vi "sub vi - Move Piezo Stage (Single).vi"(3 "frequency":dbl=0.5 min=0.0, 4 "Desired Position (um)":dbl min=0.0 format="%0.6f", 5 "Axis":u16(ring) items=["X", "Y", "Z"]) -> (0 "Z Position":dbl, 1 "Y Position":dbl, 2 "X Position":dbl)   [LabVIEW 2010]
uses:
  <vilib>/DAQmx/write.llb/DAQmx Write (Analog DBL 1Chan 1Samp).vi
  <vilib>/DAQmx/create/channels.llb/DAQmx Create Channel (AO-Voltage-Basic).vi
  <vilib>/daqmx/miscellaneous.llb/DAQmx Fill In Error Info.vi
panel:
  out "Strain2um":dbl
  # "About this Program:\n     - This program moves the piezo stage in the \n        desired axis to a desired position"
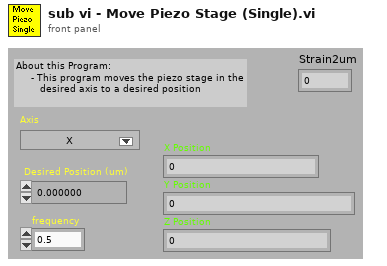
[diagram p1: front panel]
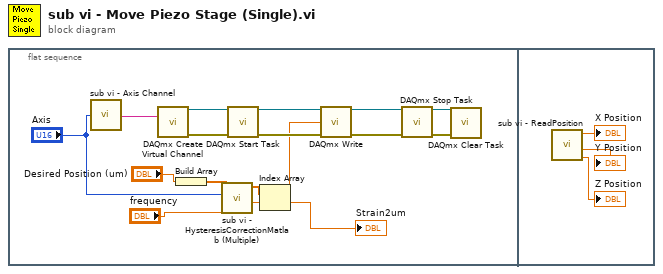
[diagram p0: block diagram]
diagram:
  n1 = flat-sequence {
    frame #0 {
      n2 = call "sub vi - Axis Channel.vi"("Axis"="Axis") -> ("physical channels"=w1:tag)
      n3 = call-poly <vilib>:"DAQmx Create Virtual Channel.vi"("physical channels"=w1) -> ("task out"=w16:refnum<k21>, "error out"=w15:errorcluster)  [unwired: 8 in, 5 out]
      n4 = Build Array("Desired Position (um)") -> (w3:dbl[])
      n5 = call "sub vi - HysteresisCorrectionMatlab (Multiple).vi"("frequency"="frequency", "Axis"="Axis", "desired positions"=w3) -> ("Strain2um"=→"Strain2um":dbl, "correctV"=w5:dbl[])  [unwired: 7 out]
      n6 = call <vilib>:"DAQmx Start Task.vi"("task/channels in"=w16, "error in"=w15) -> ("task out"=w12:refnum<k21>, "error out"=w9:errorcluster)  [unwired: 12 out]
      n7 = Index Array(array=w5) -> (element=w4:dbl)  [unwired: 1 in]
      n8 = call-poly <vilib>:"DAQmx Write.vi"("task/channels in"=w12, "data"=w4, "error in"=w9) -> ("task out"=w11:refnum<k21>, "error out"=w10:errorcluster)  [unwired: 1 in, 10 out]
      n9 = call <vilib>:"DAQmx Stop Task.vi"("task/channels in"=w11, "error in"=w10) -> ("task out"=w14:refnum<k21>, "error out"=w13:errorcluster)  [unwired: 12 out]
      n10 = call <vilib>:"DAQmx Clear Task.vi"("task in"=w14, "error in"=w13) -> ()  [unwired: 14 out]
    }
    frame #1 {
      n11 = call "sub vi - ReadPosition.vi"() -> ("Z Position"=→"Z Position":dbl, "Y Position"=→"Y Position":dbl, "X Position"=→"X Position":dbl)  [unwired: 9 out]
    }
  }
